vi "GetPixelCount.vi"(8 "error in (no error)":errorcluster, 11 "Microscope in":refnum<class "Microscope.lvclass">) -> (0 "error out":errorcluster, 1 "Grabbed all required frames?":bool, 2 "Image full":bool, 3 "Microscope out":refnum<class "Microscope.lvclass">)   [LabVIEW 2012, in "Microscope.lvclass"]
uses:
  classes/Microscope.lvclass
  classes/Microscope.lvclass/Microscope.ctl
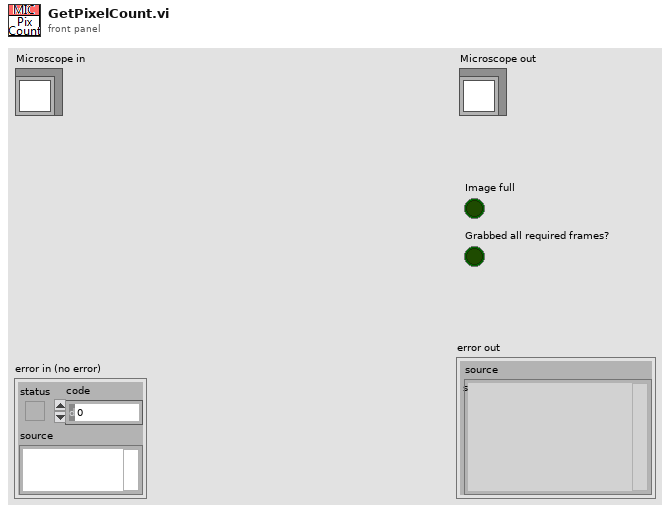
[diagram p1: front panel]
types:
  T1 = typedef "Scan Type.ctl" = enum16{"None", "Point", "Full Image Continuous", "Full Image Grab"}
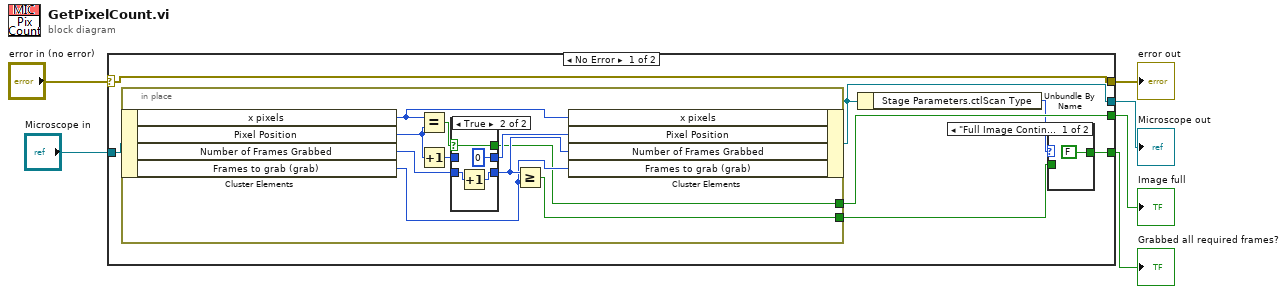
[diagram p0: block diagram]
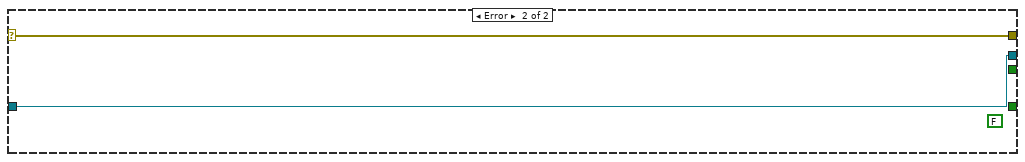
[diagram p4: hidden frame]
diagram:
  n1 = case shown="No Error" "error in (no error)" {
    selector: "error in (no error)" -> [w11 w34]
    tunnel: [w11 w34] -> w5
    tunnel: [w10 w33] -> w3
    tunnel: "Microscope in" -> [w13 w33]
    tunnel: [w12 _] -> w2
    tunnel: [w7 _] -> w1
    frame No Error {
      n2 = in-place {
        in-place-border: [w16] -> w12
        in-place-border: [w20] -> w8
        n3 = in-place-cluster #1(w13) -> ("x pixels"=w22:i32, "Pixel Position"=w18:i32, "Number of Frames Grabbed"=w23:i32, "Frames to grab (grab)"=w19:i32)
        n4 = Equal?(x=w22, y=w18) -> (x = y?=w25:bool)
        n5 = Increment(x=w18) -> (x+1=w17:i32)
        n6 = case shown="True" w25 {
          selector: w25 -> [w26 w29]
          tunnel: [w28 0] -> w24
          tunnel: w17 -> [w28 _]
          tunnel: w23 -> [w27 w31]
          tunnel: [w27 w30] -> w21
          tunnel: [w26 w29] -> w16
          frame False {
          }
          frame True {
            n7 = Increment(x=w31) -> (x+1=w30:i32)
          }
        }
        n8 = Greater Or Equal?(x=w21, y=w19) -> (x >= y?=w20:bool)
        n9 = in-place-cluster #1("x pixels"=w22, "Pixel Position"=w24, "Number of Frames Grabbed"=w21, "Frames to grab (grab)"=w19) -> (w10:refnum<class "Microscope.lvclass">)
      }
      n10 = Unbundle By Name(w10) -> ("Stage Parameters.ctlScan Type"=w9:T1)
      n11 = case shown="\"Full Image Continuous\", Default" w9 {
        tunnel: w8 -> [_ w15]
        tunnel: [FALSE w15] -> w7
        frame "Full Image Continuous", Default {
        }
        frame "Full Image Grab" {
        }
      }
    }
    frame Error {
      (unwired) FALSE ("bWait")
    }
  }
  "error out" <- w5
  "Microscope out" <- w3
  "Image full" <- w2
  "Grabbed all required frames?" <- w1
